vi "SetMainSN.vi"(11 "YTESTER测试数据":T1) -> (3 "YTESTER结论":T2)   [LabVIEW 2017]
uses:
  YtCommon.lvlibp/yt`Step StepBaseInput.ctl
  YtCommon.lvlibp/yt`Step StepResult.ctl
  YtCommon.lvlibp/yt`Step TestData.ctl
  YtCommon.lvlibp/yt`Step System Queue.ctl
  YtCommon.lvlibp
panel:
  in  "YTESTER开放参数":cluster{"YTESTER_BaseInput":T3, "赋值源":string}={"YTESTER_BaseInput"={"isTest"=FALSE, "isSkip"=FALSE, "StepName"="主SN赋值", "OnPass"=enum."Next", "OnFail"=enum."Next", "ReTestNumber"=0.0}, "赋值源"=""}
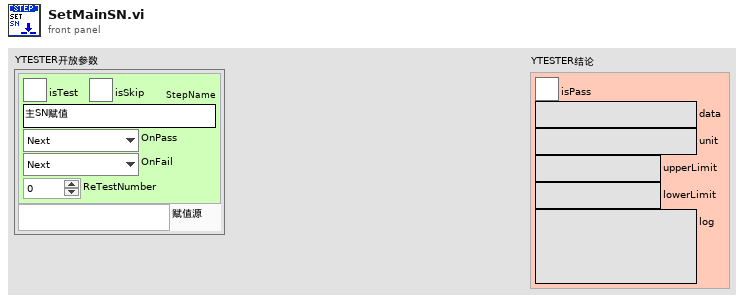
[diagram p1: front panel]
types:
  T1 = typedef "YtCommon.lvlibp/yt`Step TestData.ctl" = cluster{"Socket(From1)":i32, "SN":refnum<notifier>, "StopFlagRef":refnum<notifier>, "YT System Queue":refnum<queue>}
  T2 = typedef "YtCommon.lvlibp/yt`Step StepResult.ctl" = cluster{"isPass":bool, "data":string, "unit":string, "upperLimit":string, "lowerLimit":string, "log":string}
  T3 = typedef "YtCommon.lvlibp/yt`Step StepBaseInput.ctl" = cluster{"isTest":bool, "isSkip":bool, "StepName":string, "OnPass":enum16{"Next", "ToOVER", "Terminate"}, "OnFail":enum16{"Next", "ToOVER", "Terminate"}, "ReTestNumber":dbl}
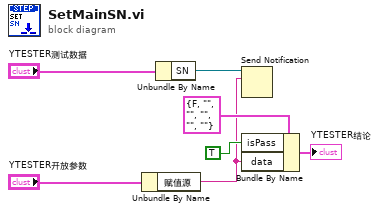
[diagram p0: block diagram]
diagram:
  n1 = Unbundle By Name("YTESTER开放参数") -> ("赋值源"=w1:string)
  n2 = Unbundle By Name("YTESTER测试数据") -> ("SN"=w3:refnum<notifier>)
  n3 = Send Notification(notification=w1, notifier=w3) -> ()  [unwired: 1 in, 2 out]
  n4 = Bundle By Name(cluster=T2 {"isPass"=FALSE, "data"="", "unit"="", "upperLimit"="", "lowerLimit"="", "log"=""} ("Result"), "isPass"=TRUE, "data"=w1) -> (→"YTESTER结论":T2)
